vi "Write SSI Encoder.vi"(10 "SSI Encoder":i32, 11 "Encoder in":refnum<class "Encoder.lvclass">) -> (3 "Encoder out":refnum<class "Encoder.lvclass">)   [LabVIEW 2013, in "Encoder.lvclass"]
uses:
  Encoder.lvclass
  Encoder.lvclass/Encoder.ctl
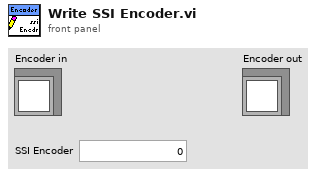
[diagram p1: front panel]
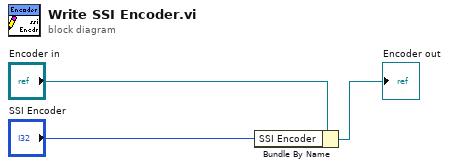
[diagram p0: block diagram]
diagram:
  n1 = Bundle By Name(cluster="Encoder in", "SSI Encoder"="SSI Encoder") -> (→"Encoder out":refnum<class "Encoder.lvclass">)
